vi "convertPhysicalChannelNames.vi"(8 "error in (no error)":errorcluster, 10 "PhysicalChannels":string, 11 "niDAQmxAO.lvclass in":refnum<class "niDAQmxAO.lvclass">) -> (0 "error out":errorcluster, 2 "channel_names":string, 3 "niDAQmxAO.lvclass out":refnum<class "niDAQmxAO.lvclass">)   [LabVIEW 2009, in "Hardware.lvlib" / "Channels.lvlib" / "niDAQmxAO.lvclass"]
uses:
  niDAQmxAO.lvclass
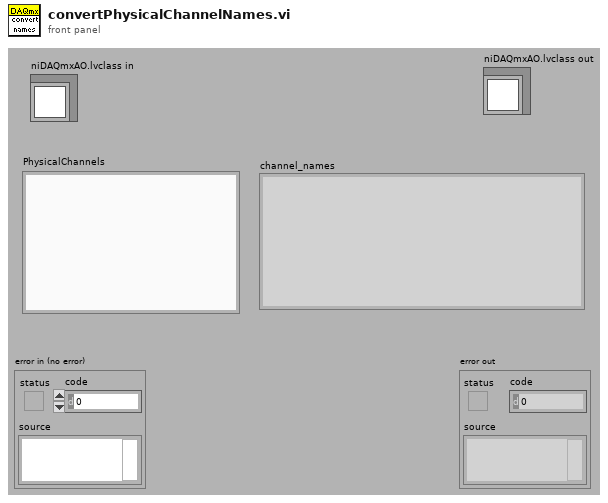
[diagram p1: front panel]
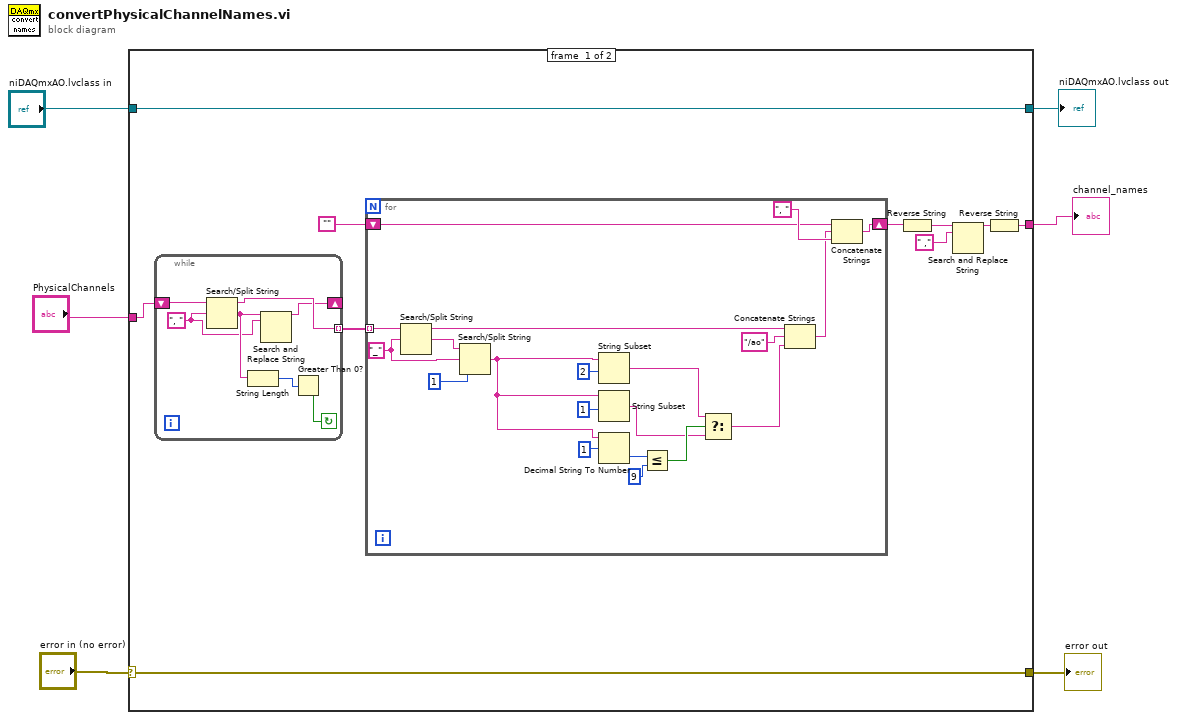
[diagram p0: block diagram]
diagram:
  n1 = case shown="No Error" "error in (no error)" {
    selector: "error in (no error)" -> [w15 w45]
    tunnel: [w15 w45] -> w5
    tunnel: [w16 w44] -> w1
    tunnel: "niDAQmxAO.lvclass in" -> [w16 w44]
    tunnel: "PhysicalChannels" -> [w14 _]
    tunnel: [w7 _] -> w3
    frame #0 {
      n2 = while {
        shift-right: [w39] -> _
        shift-left: w14 -> [w43]
        tunnel: [w42] -> w13 mode=indexing
        stop <- w37 continue-if-true
        w40 = ", "
        n3 = Search/Split String(string=w43, search string/char (-)=w40) -> (substring before match=w42:string, match + rest of string=w41:string)  [unwired: 1 in, 1 out]
        n4 = String Length(string=w41) -> (length=w38:i32)
        n5 = Search and Replace String(input string=w41, search string=w40) -> (result string=w39:string)  [unwired: 6 in, 3 out]
        n6 = Greater Than 0?(x=w38) -> (x > 0?=w37:bool)
      }
      n7 = for {
        tunnel: w13 -> [w31] mode=indexing
        shift-right: [w28] -> w8
        shift-left: "" -> [w29]
        w34 = "_"
        n8 = Search/Split String(string=w31, search string/char (-)=w34) -> (substring before match=w36:string, match + rest of string=w35:string)  [unwired: 1 in, 1 out]
        n9 = Search/Split String(string=w35, search string/char (-)=w34, offset (0)=1) -> (match + rest of string=w32:string)  [unwired: 2 out]
        n10 = String Subset(string=w32, offset (0)=2) -> (substring=w20:string)  [unwired: 1 in]
        n11 = String Subset(string=w32, offset (0)=1) -> (substring=w18:string)  [unwired: 1 in]
        n12 = Decimal String To Number(string=w32, offset=1) -> (number=w23:i32)  [unwired: 1 in, 1 out]
        n13 = Less Or Equal?(x=w23, y=9) -> (x <= y?=w21:bool)
        n14 = Select(t=w20, s=w21, f=w18) -> (s? t:f=w17:string)
        n15 = Concatenate Strings(w36, "/ao", w17) -> (w27:string)
        n16 = Concatenate Strings(w29, w27, ", ") -> (w28:string)
      }
      n17 = Reverse String(1:w8) -> (0:w11:string)
      n18 = Search and Replace String(input string=w11, search string=" ,") -> (result string=w9:string)  [unwired: 6 in, 3 out]
      n19 = Reverse String(1:w9) -> (0:w7:string)
    }
    frame #1 {
    }
  }
  "error out" <- w5
  "channel_names" <- w3
  "niDAQmxAO.lvclass out" <- w1
